vi "Get Position.vi"   [LabVIEW 2020, in "video_io.lvlib" / "Reader.lvclass"]
uses:
  Reader.lvclass
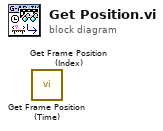
[diagram p0: block diagram]
diagram:
  n1 = call "Get Frame Position (Time).vi"() -> ()  [unwired: 9 in, 3 out]
  n2 = call "Get Frame Position (Index).vi"() -> ()  [unwired: 9 in, 3 out]
